vi "Schmitt Trigger Demo.vi"() -> ()   [LabVIEW 2013]
panel:
  out "inv out":bool
  out "out":bool
  in  "lo":dbl(knob) scale=0.0..10.0
  in  "in":dbl(knob) scale=0.0..10.0
  in  "hi":dbl(knob) scale=0.0..10.0
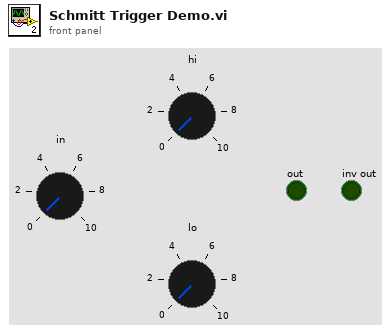
[diagram p1: front panel]
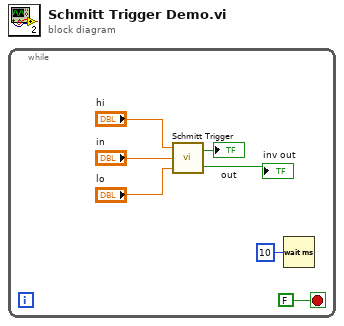
[diagram p0: block diagram]
diagram:
  n1 = while {
    stop <- FALSE stop-if-true
    n2 = call "Schmitt Trigger.vi"("lo"="lo", "in"="in", "hi"="hi") -> ("inv out"=→"inv out":bool, "out"=→"out":bool)
    n3 = Wait (ms)(milliseconds to wait=u32 10) -> ()  [unwired: 1 out]
  }
